vi "action.vi"(0 "HGF_ThreadTask":refnum<class "HGF_ThreadTask.lvclass">, 5 "error in (no error)":errorcluster, 8 "HGF_ThreadWorker":refnum<class "HGF_ThreadWorker.lvclass">) -> (10 "dup HGF_ThreadWorker":refnum<class "HGF_ThreadWorker.lvclass">, 14 "dup HGF_ThreadTask":refnum<class "HGF_ThreadTask.lvclass">, 19 "error out":errorcluster)   [LabVIEW 2014, in "HGF_BaseClasses.lvlib" / "HGF_ThreadTask.lvclass"]
uses:
  HGF_ThreadTask.lvclass
  HGF_Auxiliary/HGF_Auxiliary.lvlib
  HGF_Auxiliary/ErrorCode.ctl
  HGF_Auxiliary/Severity.ctl
  HGF_ThreadWorker/HGF_ThreadWorker.lvclass
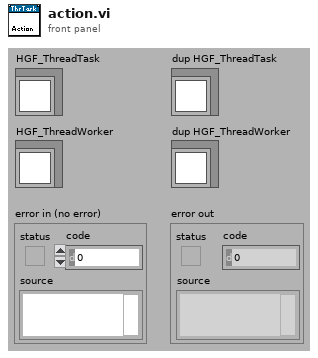
[diagram p1: front panel]
types:
  T1 = typedef "HGF_Auxiliary.lvlib/Severity.ctl" = enum16{"Info", "Warning", "Fault", "Error", "Fatal"}
  T2 = typedef "HGF_Auxiliary.lvlib/ErrorCode.ctl" = enum32{"No error", "Function not supported.", "This VI is for friends only.", "Reference object aready exisits.", "Parameter out of range.", "Not a rendezvous.", "Invalid notifier reference.", "Invalid queue reference.", "Self-Test not supported.", "Reset not supported.", "IDN query not supported.", "Error query not supported.", "Incorrect addressee.", "Object already exists.", "No class name specified", "Driver not supported", "Attribute is not writable"}
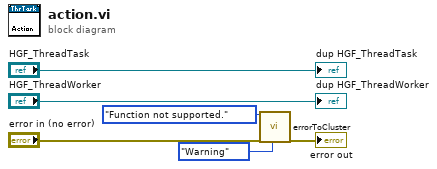
[diagram p0: block diagram]
diagram:
  n1 = call "errorToCluster.vi"("error code"=ErrorCode."Function not supported.", "error in (no error)"="error in (no error)", "severity (Error)"=Severity."Warning") -> ("error out"=→"error out":errorcluster)  [unwired: 2 in, 14 out]
  "dup HGF_ThreadTask" <- "HGF_ThreadTask"
  "dup HGF_ThreadWorker" <- "HGF_ThreadWorker"
